vi "KE622x -- 2182 -A Get Range tmp.vi"(0 "622x Resource In":refnum<visa-resource-name>, 1 "Check For SCPI Errors? (T)":bool=TRUE, 11 "error in (no error)":errorcluster) -> (4 "622x Resource Out (dupl)":refnum<visa-resource-name>, 8 "2182/2182A Range":T1, 15 "error out":errorcluster)   [LabVIEW 2014, in "Keithley 622x tmp.lvlib"]
uses:
  Keithley 622x tmp.lvlib
  Typedefs/KE2182 -- Voltage Ranges.ctl
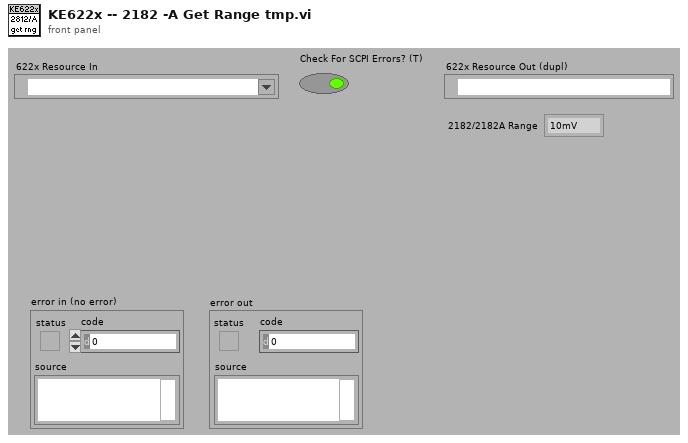
[diagram p1: front panel]
types:
  T1 = typedef "Keithley 622x tmp.lvlib/KE2182 -- Voltage Ranges.ctl" = enum16{"10mV", "100mV", "1V", "10V", "100V"}
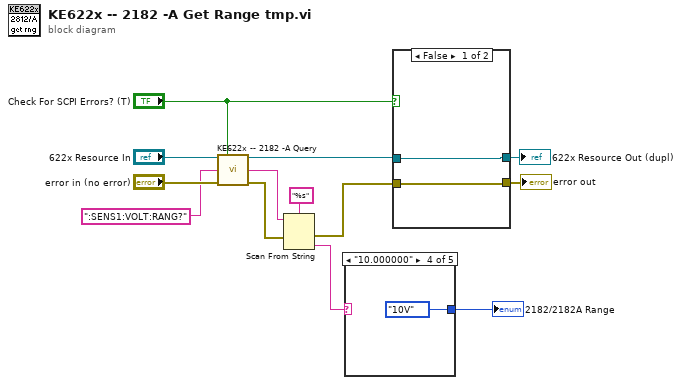
[diagram p0: block diagram]
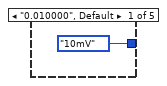
[diagram p2: hidden frame]
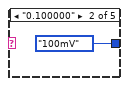
[diagram p3: hidden frame]
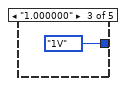
[diagram p4: hidden frame]
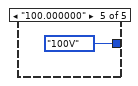
[diagram p5: hidden frame]
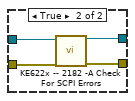
[diagram p6: hidden frame]
diagram:
  n1 = call "KE622x -- 2182 -A Query.vi"("622x Resource In"="622x Resource In", "Check For SCPI Errors? (T)"="Check For SCPI Errors? (T)", "2182-A Write String"=":SENS1:VOLT:RANG?", "error in (no error)"="error in (no error)") -> ("622x Resource Out (dupl)"=w7:refnum<visa-resource-name>, "2182-A Reponse String"=w8:string, "error out"=w10:errorcluster)  [unwired: 9 in]
  n2 = Scan From String(format string="%s", input string=w8, error in=w10) -> (error out=w6:errorcluster, output 1=w2:string)  [unwired: 2 in, 2 out]
  n3 = case shown="\"10.000000\"" w2 {
    tunnel: [KE2182_--_Voltage_Ranges."10mV" ("2182/2182A Range") KE2182_--_Voltage_Ranges."100mV" ("2182/2182A Range") KE2182_--_Voltage_Ranges."1V" ("2182/2182A Range") KE2182_--_Voltage_Ranges."10V" ("2182/2182A Range") KE2182_--_Voltage_Ranges."100V" ("2182/2182A Range")] -> w1
    frame "0.010000", Default {
    }
    frame "0.100000" {
    }
    frame "1.000000" {
    }
    frame "10.000000" {
    }
    frame "100.000000" {
    }
  }
  "2182/2182A Range" <- w1
  n4 = case shown="False" "Check For SCPI Errors? (T)" {
    tunnel: w7 -> [w20 w24]
    tunnel: w6 -> [w19 w23]
    tunnel: [w20 w22] -> w4
    tunnel: [w19 w21] -> w3
    frame False {
    }
    frame True {
      n5 = call "KE622x -- 2182 -A Check For SCPI Errors.vi"("VISA Resource In"=w24, "error in (no error)"=w23) -> ("VISA Resource Out (dupl)"=w22:refnum<visa-resource-name>, "error out"=w21:errorcluster)  [unwired: 10 in, 2 out]
    }
  }
  "622x Resource Out (dupl)" <- w4
  "error out" <- w3
